vi "XIPIN_Tri_Mode_Ethernet_MAC_9_0.vi"   [LabVIEW 2017]
doc: "The TEMAC Block LogiCORE(TM) is designed to the IEEE 802.3-2008 standard specification and supports full/half duplex operation at 10/100/1000Mbps speeds and a full duplex only operation at 2.5Gbps. In addition, it provides support for VLAN and JUMBO frames, as well as network management options such as statistics gathering and flow control. The core can be configured and monitored through an AXI interface, providing users with the flexibility to select the processor best suited to their specific application. The standalone core provides either a Gigabit Media Independent Interface (GMII) or a Reduced Gigabit Media Independent Interface (RGMII), both of which can carry Ethernet traffic at all three speeds and are suitable for connection to all industry standard PHYs of all media types. In addition, the core seamlessly interfaces to the Ethernet 1000BASE-X PCS/PMA or SGMII LogiCORE which can provide a Serial-GMII (SGMII) or can alternatively extend the functionality of the core to provide a 1000BASE-X PCS/PMA (1Gb/s and 2.5Gb/s Optical PHY Standard) creating a complete Gig/2.5GigE MAC core solution.\n------------------------------------\n<b>Need License</b> : Yes\n<b>Interface</b> : AXI4 AXI4-Stream"
uses:
  <vilib>/rvi/XilinxIP/XIPIN_XNode/niFpgaXIPIN.xnode
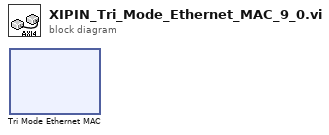
[diagram p0: block diagram]
diagram:
  n1 = xnode ("Tri Mode Ethernet MAC")() -> ()
